vi "PreInstall.vi"(10 "Variant":variant) -> (0 "error out":errorcluster)   [LabVIEW 2012]
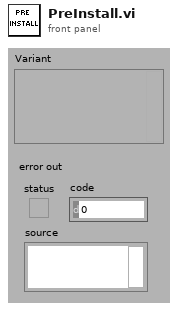
[diagram p1: front panel]
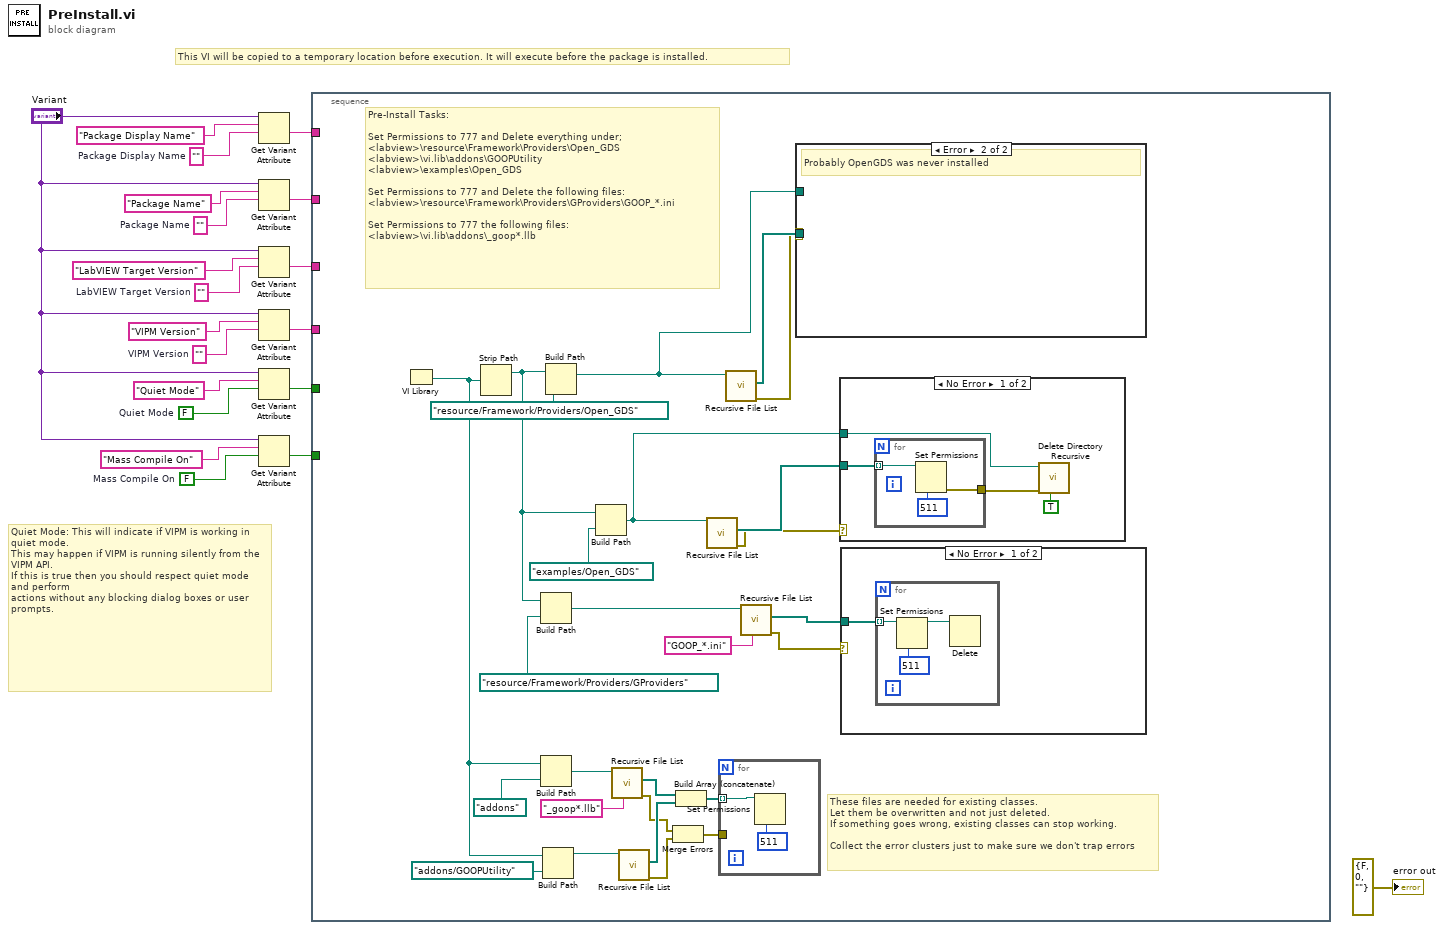
[diagram p0: block diagram]
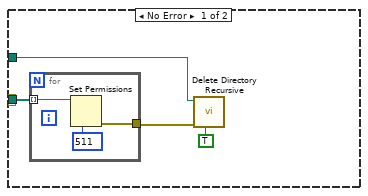
[diagram p3: hidden frame]
diagram:
  w1 = FALSE  # Mass Compile On
  w3 = ""  # Package Display Name
  w10 = FALSE  # Quiet Mode
  w13 = ""  # VIPM Version
  w15 = ""  # LabVIEW Target Version
  w17 = ""  # Package Name
  # "Quiet Mode: This will indicate if VIPM is working in quiet mode.\nThis may happen if VIPM is running silently from the VIPM API.\nIf this is true then you should respect quiet mode and perform\nactions without any blocking dialog boxes or user prompts."
  # "This VI will be copied to a temporary location before execution. It will execute before the package is installed."
  n1 = Get Variant Attribute(Variant="Variant", name="Package Display Name", default value (empty Variant)=w3) -> (value=w9:string)  [unwired: 1 in, 3 out]
  n2 = Get Variant Attribute(Variant="Variant", name="Package Name", default value (empty Variant)=w17) -> (value=w8:string)  [unwired: 1 in, 3 out]
  n3 = Get Variant Attribute(Variant="Variant", name="LabVIEW Target Version", default value (empty Variant)=w15) -> (value=w7:string)  [unwired: 1 in, 3 out]
  n4 = Get Variant Attribute(Variant="Variant", name="VIPM Version", default value (empty Variant)=w13) -> (value=w6:string)  [unwired: 1 in, 3 out]
  n5 = Get Variant Attribute(Variant="Variant", name="Quiet Mode", default value (empty Variant)=w10) -> (value=w5:bool)  [unwired: 1 in, 3 out]
  n6 = Get Variant Attribute(Variant="Variant", name="Mass Compile On", default value (empty Variant)=w1) -> (value=w4:bool)  [unwired: 1 in, 3 out]
  n7 = stacked-sequence {
    tunnel: w9 -> [_]
    tunnel: w8 -> [_]
    tunnel: w7 -> [_]
    tunnel: w6 -> [_]
    tunnel: w5 -> [_]
    tunnel: w4 -> [_]
    frame #0 {
      # "These files are needed for existing classes.\nLet them be overwritten and not just deleted.\nIf something goes wrong, existing classes can stop working.\n\nCollect the error clusters just to make sure we don't trap errors"
      # "Pre-Install Tasks:\n\nSet Permissions to 777 and Delete everything under;\n<labview>\\resource\\Framework\\Providers\\Open_GDS\n<labview>\\vi.lib\\addons\\GOOPUtility\n<labview>\\examples\\Open_GDS\n\nSet Permissions to 777 and Delete the following files:\n<labview>\\resource\\Framework\\Providers\\GProviders\\GOOP_*.ini\n\nSet Permissions to 777 the following files:\n<labview>\\vi.lib\\addons\\_goop*.llb"
      n8 = VI Library() -> (path=w36:path)
      n9 = Strip Path(path=w36) -> (stripped path=w42:path)  [unwired: 1 out]
      n10 = Build Path(base path=w42, name or relative path=path "resource/Framework/Providers/GProviders" ("path")) -> (appended path=w41:path)
      n11 = Build Path(base path=w36, name or relative path=path "addons" ("path")) -> (appended path=w37:path)
      n12 = Build Path(base path=w36, name or relative path=path "addons/GOOPUtility" ("path")) -> (appended path=w31:path)
      n13 = Build Path(base path=w42, name or relative path=path "resource/Framework/Providers/Open_GDS" ("path")) -> (appended path=w30:path)
      n14 = Build Path(base path=w42, name or relative path=path "examples/Open_GDS" ("path")) -> (appended path=w28:path)
      n15 = call <vilib>:"Recursive File List.vi"("pattern"="_goop*.llb", "Folder Path"=w37) -> ("error out"=w23:errorcluster, "All Files in Dir"=w33:path[])  [unwired: 5 in, 3 out]
      n16 = call <vilib>:"Recursive File List.vi"("Folder Path"=w31) -> ("error out"=w22:errorcluster, "All Files in Dir"=w34:path[])  [unwired: 6 in, 3 out]
      n17 = Merge Errors(w23, w22) -> (w21:errorcluster)
      n18 = Build Array (concatenate)(w33, w34) -> (w32:path[])
      n19 = call <vilib>:"Recursive File List.vi"("Folder Path"=w28) -> ("error out"=w26:errorcluster, "All Files in Dir"=w27:path[])  [unwired: 6 in, 3 out]
      n20 = for {
        tunnel: w32 -> [w65] mode=indexing
        tunnel: w21 -> [_]
        n21 = Set Permissions(7:i16 511 ("permissions"), 11:w65) -> ()  [unwired: 3 in, 2 out]
      }
      n22 = call <vilib>:"Recursive File List.vi"("Folder Path"=w30) -> ("error out"=w25:errorcluster, "All Files in Dir"=w29:path[])  [unwired: 6 in, 3 out]
      n23 = call <vilib>:"Recursive File List.vi"("pattern"="GOOP_*.ini", "Folder Path"=w41) -> ("error out"=w24:errorcluster, "All Files in Dir"=w39:path[])  [unwired: 5 in, 3 out]
      n24 = case shown="Error" w25 {
        tunnel: w30 -> [w53 _]
        tunnel: w29 -> [w51 _]
        frame No Error {
          n25 = for {
            tunnel: w51 -> [w57] mode=indexing
            tunnel: [w55] -> w52
            n26 = Set Permissions(7:i16 511 ("permissions"), 11:w57) -> (0:w55:errorcluster)  [unwired: 3 in, 1 out]
          }
          n27 = call <vilib>:"Delete Directory Recursive.vi"("keep deleting on error? (F)"=TRUE, "error in (no error)"=w52, "Folder to Delete"=w53) -> ()  [unwired: 7 in, 2 out]
        }
        frame Error {
          # "Probably OpenGDS was never installed"
        }
      }
      n28 = case shown="No Error" w26 {
        tunnel: w28 -> [w61 _]
        tunnel: w27 -> [w58 _]
        frame No Error {
          n29 = for {
            tunnel: w58 -> [w64] mode=indexing
            tunnel: [w62] -> w59
            n30 = Set Permissions(7:i16 511 ("permissions"), 11:w64) -> (0:w62:errorcluster)  [unwired: 3 in, 1 out]
          }
          n31 = call <vilib>:"Delete Directory Recursive.vi"("keep deleting on error? (F)"=TRUE, "error in (no error)"=w59, "Folder to Delete"=w61) -> ()  [unwired: 7 in, 2 out]
        }
        frame Error {
          # "Probably OpenGDS was never installed"
        }
      }
      n32 = case shown="No Error" w24 {
        tunnel: w39 -> [w47 _]
        frame No Error {
          n33 = for {
            tunnel: w47 -> [w48] mode=indexing
            n34 = Set Permissions(7:i16 511 ("permissions"), 11:w48) -> (3:w50:path)  [unwired: 3 in, 1 out]
            n35 = Delete(path (use dialog)=w50) -> ()  [unwired: 4 in, 3 out]
          }
        }
        frame Error {
          # "Probably OpenGDS was not installed"
        }
      }
    }
  }
  "error out" <- errorcluster {"status"=FALSE, "code"=0, "source"=""} ("error out")
